vi "ReadControlMode.vi"(8 "error in (no error)":errorcluster, 11 "Hardware Resources in":T1) -> (0 "error out":errorcluster, 2 "number":u32, 3 "Hardware Resources out":T1)   [LabVIEW 2016]
uses:
  Hardware Configuration.ctl
  <vilib>/NI Modbus.llb/MB Serial Master Query Read Coils (poly).vi
  Acquisition.lvlib
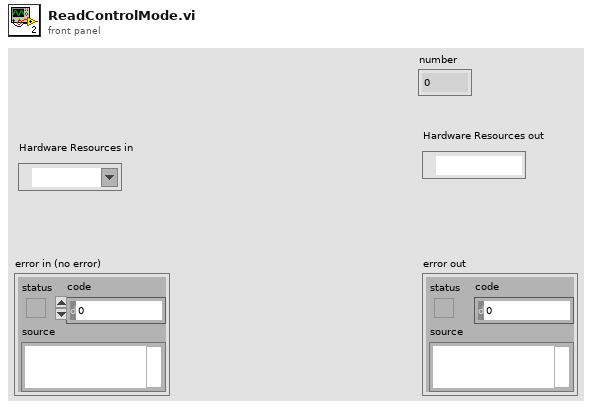
[diagram p1: front panel]
types:
  T1 = typedef "Acquisition.lvlib/Hardware Configuration.ctl" = refnum<visa-resource-name>
  T2 = cluster{"Mode":enum16{"RTU", "ASCII"}, "Slave Address":u8}
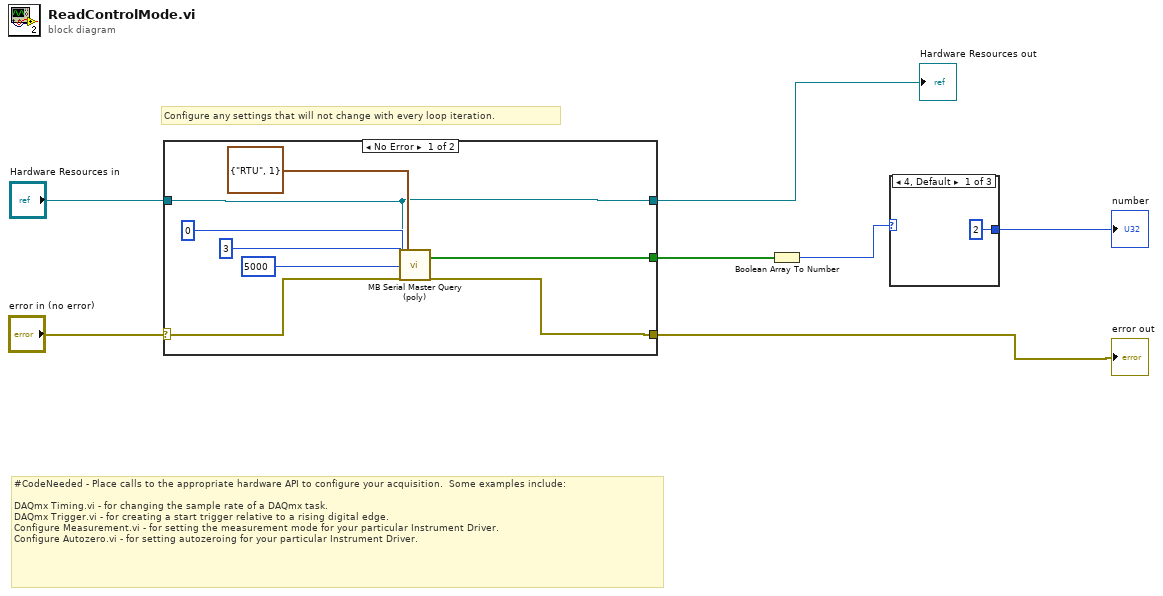
[diagram p0: block diagram]
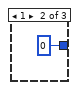
[diagram p2: hidden frame]
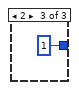
[diagram p3: hidden frame]
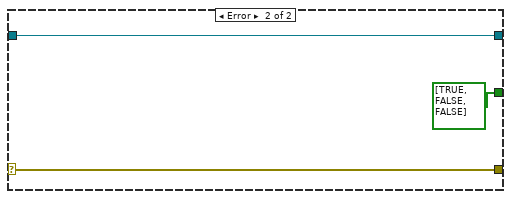
[diagram p4: hidden frame]
diagram:
  # "Configure any settings that will not change with every loop iteration."
  # "#CodeNeeded - Place calls to the appropriate hardware API to configure your acquisition.  Some examples include:\n\nDAQmx Timing.vi - for changing the sample rate of a DAQmx task.\nDAQmx Trigger.vi - for creating a start trigger relative to a rising digital edge.\nConfigure Measurement.vi - for setting the measurement mode for your particular Instrument Driver.\nConfigure Autozero.vi - for setting autozeroing for your particular Instrument Driver."
  n1 = case shown="No Error" "error in (no error)" {
    selector: "error in (no error)" -> [w14 w17]
    tunnel: [w15 w17] -> w4
    tunnel: "Hardware Resources in" -> [w8 w18]
    tunnel: [w8 w18] -> w5
    tunnel: [w9 bool[] [TRUE, FALSE, FALSE] ("Coils")] -> w3
    frame No Error {
      n2 = call-poly <vilib>:"MB Serial Master Query (poly).vi"("VISA resource name"=w8, "Starting Address"=u16 0, "Quantity"=u16 3, "Timeout"=u32 5000, "error in"=w14, "Serial Parameters"=T2 {"Mode"=enum."RTU", "Slave Address"=1}) -> ("Coils"=w9:bool[], "error out"=w15:errorcluster)  [unwired: 10 in, 2 out]
    }
    frame Error {
    }
  }
  "Hardware Resources out" <- w5
  "error out" <- w4
  n3 = Boolean Array To Number(Boolean array=w3) -> (number=w2:u32)
  n4 = case shown="4, Default" w2 {
    tunnel: [u32 2 u32 0 u32 1] -> w1
    frame 4, Default {
    }
    frame 1 {
    }
    frame 2 {
    }
  }
  "number" <- w1
